vi "Tetra_BPF.vi"(0 "COMPORT":refnum<visa-resource-name>="COM4", 3 "Rev-C(t)":bool=TRUE, 4 "ant-port":i32=2 min=0 max=12 step=1, 5 "error in (no error)":errorcluster, 6 "RO(t)":bool, 7 "RX/TX":i32(ring)=1 items=["RX", "TX"], 9 "bpf(sel)":i32(ring)=2 items=["HIGH", "LOW"], 11 "Open Ser(t)":bool, 12 "milliseconds to wait":u32, 13 "Close Ser(t)":bool) -> (10 "bpf":i32=1, 14 "comport":refnum<visa-resource-name>="COM4", 19 "error out":errorcluster)   [LabVIEW 2018]
panel:
  out "rx?(t)":bool
  out "cmd":string
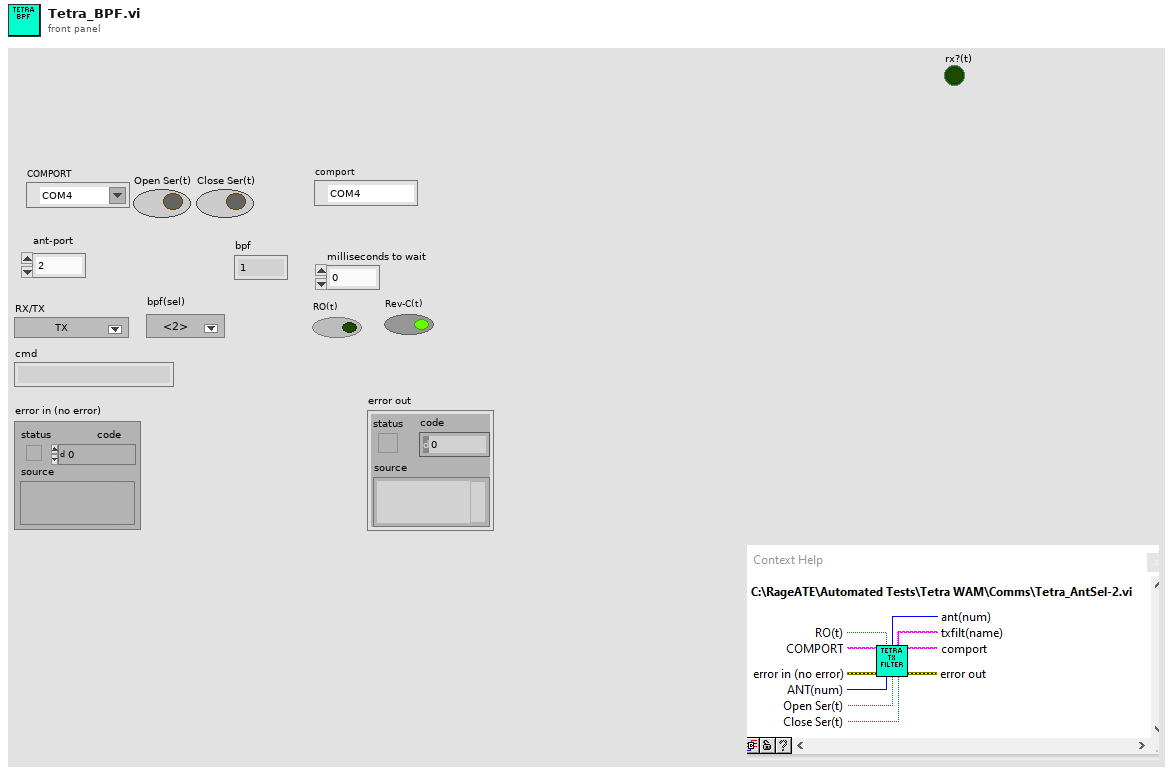
[diagram p1: front panel]
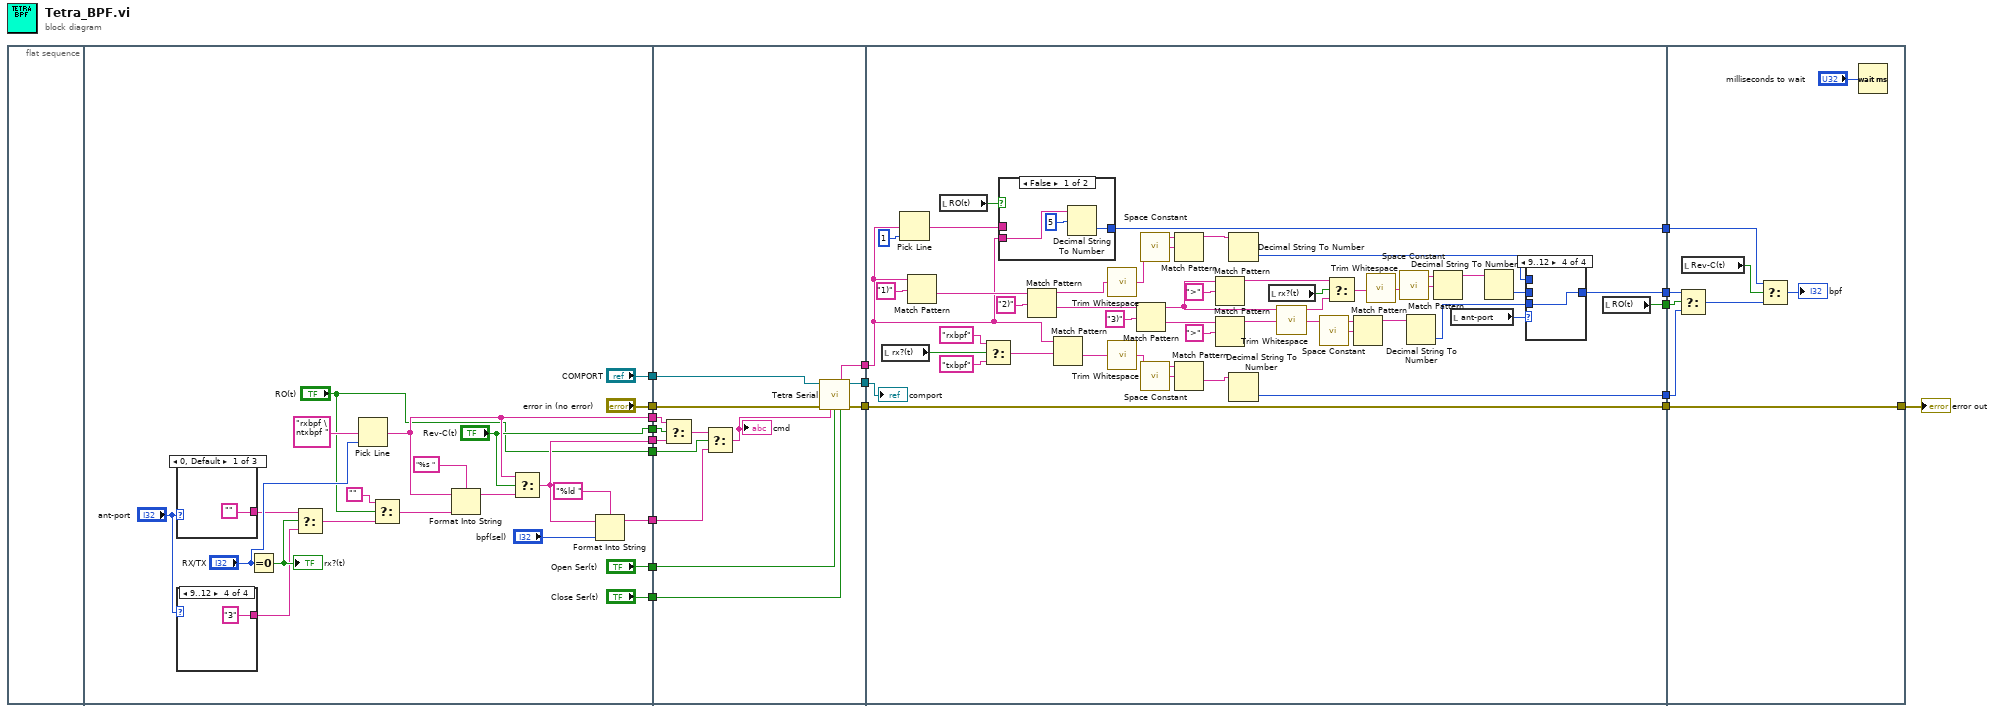
[diagram p0: block diagram]
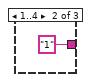
[diagram p2: hidden frame]
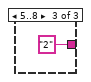
[diagram p3: hidden frame]
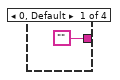
[diagram p4: hidden frame]
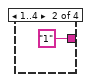
[diagram p5: hidden frame]
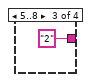
[diagram p6: hidden frame]
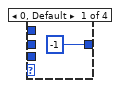
[diagram p7: hidden frame]
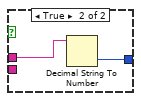
[diagram p10: hidden frame]
diagram:
  n1 = flat-sequence {
    tunnel: ["error in (no error)"] -> w18
    tunnel: ["COMPORT"] -> w17
    tunnel: [w37] -> w16
    tunnel: ["Open Ser(t)"] -> w15
    tunnel: [w27] -> w14
    tunnel: ["Close Ser(t)"] -> w13
    tunnel: ["RO(t)"] -> w10
    tunnel: [w24] -> w6
    tunnel: ["Rev-C(t)"] -> w5
    tunnel: w18 -> [w61]
    tunnel: w17 -> [w60]
    tunnel: w16 -> [w54]
    tunnel: w15 -> [w59]
    tunnel: w14 -> [w53]
    tunnel: w13 -> [w56]
    tunnel: [w58] -> w12
    tunnel: [w57] -> w11
    tunnel: w10 -> [w50]
    tunnel: [w55] -> w9
    tunnel: w6 -> [w51]
    tunnel: w5 -> [w49]
    tunnel: w9 -> [w72]
    tunnel: w11 -> [w105]
    tunnel: w12 -> [w103]
    tunnel: [w103] -> w8
    tunnel: [w92] -> w4
    tunnel: [w90] -> w3
    tunnel: [w63] -> w2
    tunnel: [w62] -> w1
    tunnel: w8 -> [w124]
    tunnel: [w124] -> w7
    tunnel: w4 -> [w122]
    tunnel: w3 -> [w119]
    tunnel: w2 -> [w117]
    tunnel: w1 -> [w116]
    frame #0 {
    }
    frame #1 {
      n2 = case shown="0, Default" "ant-port" {
        tunnel: ["" "1" "2"] -> w29
        frame 0, Default {
        }
        frame 1..4 {
        }
        frame 5..8 {
        }
      }
      n3 = case shown="9..12" "ant-port" {
        tunnel: ["" "1" "2" "3"] -> w28
        frame 0, Default {
        }
        frame 1..4 {
        }
        frame 5..8 {
        }
        frame 9..12 {
        }
      }
      n4 = Equal To 0?(x="RX/TX") -> (x = 0?=w31:bool)
      "rx?(t)" <- w31
      n5 = Select(t=w29, s=w31, f=w28) -> (s? t:f=w21:string)
      n6 = Pick Line(multi-line string="rxbpf \ntxbpf ", line index="RX/TX") -> (output string=w27:string)  [unwired: 1 in]
      n7 = Select(t="", s="RO(t)", f=w21) -> (s? t:f=w20:string)
      n8 = Format Into String(format string="%s ", initial string=w27, w20) -> (resulting string=w25:string)  [unwired: 1 in, 1 out]
      n9 = Select(t=w27, s="Rev-C(t)", f=w25) -> (s? t:f=w24:string)
      n10 = Format Into String(format string="%ld ", initial string=w24, "bpf(sel)") -> (resulting string=w37:string)  [unwired: 1 in, 1 out]
    }
    frame #2 {
      n11 = Select(t=w53, s=w49, f=w51) -> (s? t:f=w52:string)
      n12 = Select(t=w52, s=w50, f=w54) -> (s? t:f=w48:string)
      "cmd" <- w48
      n13 = call "Tetra Serial.vi"("COMPORT"=w60, "error in (no error)"=w61, "Command"=w48, "Open Ser(t)"=w59, "Close Ser(t)"=w56) -> ("output"=w55:string, "comport"=w57:refnum<visa-resource-name>, "error out"=w58:errorcluster)  [unwired: 6 in, 2 out]
    }
    frame #3 {
      n14 = local read "rx?(t)"() -> (w71:bool)
      n15 = Pick Line(multi-line string=w72, line index=1) -> (output string=w102:string)  [unwired: 1 in]
      n16 = Match Pattern(string=w72, regular expression="1)") -> (after substring=w86:string)  [unwired: 1 in, 3 out]
      n17 = local read "RO(t)"() -> (w104:bool)
      n18 = Select(t="rxbpf" ("regular expression"), s=w71, f="txbpf" ("regular expression")) -> (s? t:f=w68:string)
      n19 = case shown="False" w104 {
        tunnel: w102 -> [_ w115]
        tunnel: [w112 w114] -> w92
        tunnel: w72 -> [w113 _]
        frame False {
          n20 = Decimal String To Number(string=w113, offset=5) -> (number=w112:i32)  [unwired: 1 in, 1 out]
        }
        frame True {
          n21 = Decimal String To Number(string=w115) -> (number=w114:i32)  [unwired: 2 in, 1 out]
        }
      }
      n22 = Match Pattern(string=w86, regular expression="2)") -> (before substring=w85:string, after substring=w83:string)  [unwired: 1 in, 2 out]
      n23 = Match Pattern(string=w72, regular expression=w68) -> (after substring=w67:string)  [unwired: 1 in, 3 out]
      n24 = call <vilib>:"Trim Whitespace.vi"("string"=w85) -> ("trimmed string"=w100:string)  [unwired: 1 in]
      n25 = call <vilib>:"Trim Whitespace.vi"("string"=w67) -> ("trimmed string"=w66:string)  [unwired: 1 in]
      n26 = Match Pattern(string=w83, regular expression="3)") -> (before substring=w73:string, after substring=w81:string)  [unwired: 1 in, 2 out]
      n27 = call <vilib>:"Space Constant.vi"() -> ("String"=w101:string)
      n28 = call <vilib>:"Space Constant.vi"() -> ("String"=w65:string)
      n29 = Match Pattern(string=w100, regular expression=w101) -> (before substring=w84:string)  [unwired: 1 in, 3 out]
      n30 = Match Pattern(string=w66, regular expression=w65) -> (after substring=w64:string)  [unwired: 1 in, 3 out]
      n31 = Match Pattern(string=w73, regular expression=">") -> (before substring=w76:string)  [unwired: 1 in, 3 out]
      n32 = Match Pattern(string=w81, regular expression=">") -> (before substring=w80:string)  [unwired: 1 in, 3 out]
      n33 = Decimal String To Number(string=w84) -> (number=w89:i32)  [unwired: 2 in, 1 out]
      n34 = Decimal String To Number(string=w64) -> (number=w62:i32)  [unwired: 2 in, 1 out]
      n35 = local read "rx?(t)"() -> (w74:bool)
      n36 = call <vilib>:"Trim Whitespace.vi"("string"=w80) -> ("trimmed string"=w94:string)  [unwired: 1 in]
      n37 = call <vilib>:"Space Constant.vi"() -> ("String"=w95:string)
      n38 = Select(t=w76, s=w74, f=w73) -> (s? t:f=w75:string)
      n39 = Match Pattern(string=w94, regular expression=w95) -> (before substring=w78:string)  [unwired: 1 in, 3 out]
      n40 = call <vilib>:"Trim Whitespace.vi"("string"=w75) -> ("trimmed string"=w97:string)  [unwired: 1 in]
      n41 = call <vilib>:"Space Constant.vi"() -> ("String"=w96:string)
      n42 = Decimal String To Number(string=w78) -> (number=w87:i32)  [unwired: 2 in, 1 out]
      n43 = Match Pattern(string=w97, regular expression=w96) -> (before substring=w79:string)  [unwired: 1 in, 3 out]
      n44 = local read "ant-port"() -> (w91:i32)
      n45 = Decimal String To Number(string=w79) -> (number=w88:i32)  [unwired: 2 in, 1 out]
      n46 = case shown="9..12" w91 {
        tunnel: [-1 w108 w109 w110] -> w90
        tunnel: w89 -> [_ w108 _ _]
        tunnel: w88 -> [_ _ w109 _]
        tunnel: w87 -> [_ _ _ w110]
        frame 0, Default {
        }
        frame 1..4 {
        }
        frame 5..8 {
        }
        frame 9..12 {
        }
      }
      n47 = local read "RO(t)"() -> (w63:bool)
      "comport" <- w105
    }
    frame #4 {
      n48 = Select(t=w119, s=w117, f=w116) -> (s? t:f=w118:i32)
      n49 = local read "Rev-C(t)"() -> (w120:bool)
      n50 = Select(t=w122, s=w120, f=w118) -> (s? t:f=→"bpf":i32)
      n51 = Wait (ms)(milliseconds to wait="milliseconds to wait") -> ()  [unwired: 1 out]
    }
  }
  "error out" <- w7
